vi "aoc-2025-d03-1.vi"() -> ()   [LabVIEW 2020]
panel:
  out "numbers":i32[](array[numeric])
  out "sum":i32
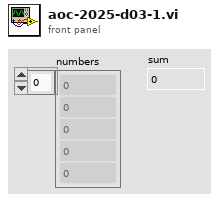
[diagram p1: front panel]
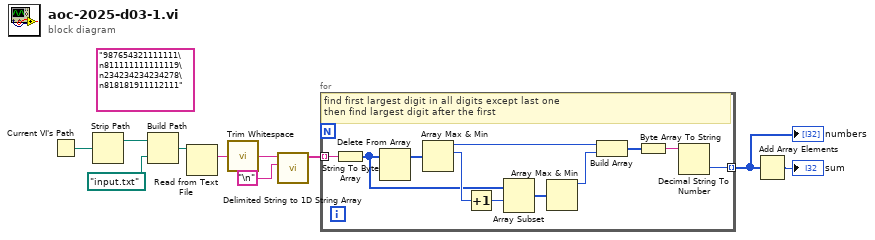
[diagram p0: block diagram]
diagram:
  (unwired) "987654321111111\n811111111111119\n234234234234278\n818181911112111"
  n1 = Current VI's Path() -> (path=w7:path)
  n2 = Strip Path(path=w7) -> (stripped path=w6:path)  [unwired: 1 out]
  n3 = Build Path(base path=w6, name or relative path=path "input.txt") -> (appended path=w4:path)
  n4 = Read from Text File(file (use dialog)=w4) -> (text=w3:string)  [unwired: 3 in, 3 out]
  n5 = call <vilib>:"Trim Whitespace.vi"("string"=w3) -> ("trimmed string"=w2:string)  [unwired: 1 in]
  n6 = call <vilib>:"Delimited String to 1D String Array.vi"("delimiter"="\n", "delimited string"=w2) -> ("string array"=w1:string[])  [unwired: 9 in]
  n7 = for {
    tunnel: w1 -> [w21] mode=indexing
    tunnel: [w14] -> w8 mode=indexing
    # "find first largest digit in all digits except last one\nthen find largest digit after the first"
    n8 = String To Byte Array(string=w21) -> (unsigned byte array=w13:u8[])
    n9 = Delete From Array(array=w13) -> (array with subset deleted=w12:u8[])  [unwired: 2 in, 1 out]
    n10 = Array Max & Min(array=w12) -> (max value=w17:u8, max index (indices)=w20:i32)  [unwired: 2 out]
    n11 = Increment(x=w20) -> (x+1=w11:i32)
    n12 = Array Subset(array=w13, index=w11) -> (w19:u8[])  [unwired: 1 in]
    n13 = Array Max & Min(array=w19) -> (max value=w18:u8)  [unwired: 3 out]
    n14 = Build Array(w17, w18) -> (w16:u8[])
    n15 = Byte Array To String(unsigned byte array=w16) -> (string=w15:string)
    n16 = Decimal String To Number(string=w15) -> (number=w14:i32)  [unwired: 2 in, 1 out]
  }
  "numbers" <- w8
  n17 = Add Array Elements(numeric array=w8) -> (sum=→"sum":i32)
